vi "TLB Native Dynamic Events ver 0.13.vi"() -> ()   [LabVIEW 2018]
uses:
  Labview Training Phase 2/Enum Controls/States for Action Engine.ctl
  TLB Type Definitions/State Type Definitions, for 0.26g versions and later 2.ctl
  TLB Type Definitions/Intruction Type Definitions.ctl
  TLB Type Definitions/Encoder cluster.ctl
  Experimental VI's/Archived VI's/MOTOR CONTROL NO PID Type Def.ctl
  Underlying VI's/I2C Master VI/I2C MASTER Type Def.ctl
  TLB Type Definitions/PING CLUSTER.ctl
  <vilib>/Studica/Studica Toolkit/NavX/NavX.lvlib
  <vilib>/Studica/Studica Toolkit/Background/DIO Channel.ctl
  Underlying VI's/NavX VI/navX type def.ctl
  <vilib>/myRIO/Instrument Drivers/Utilities/Utilities.lvlib
  <vilib>/Studica/Studica Toolkit/Background/I2C Channel.ctl
  Underlying VI's/I2C Master VI/I2C_MASTER_WRITE_NEW Type Def.ctl
  <vilib>/Studica/Studica Toolkit/NavX/TypeDefs/Flags/Z900_navX_Flags_CalibrationStatusTypeDef.ctl
  <vilib>/Studica/Studica Toolkit/NavX/TypeDefs/Flags/Z900_navX_Flags_OpStatusTypeDef.ctl
panel:
  in  "Latch":bool
  in  "y Stepper value":u8
  out "Arduino Data":T1
  in  "Arduino mode":T2
  out "Detect?":bool
  out "Status":T5 {"OP Status" items=["INITIALIZING", "SELFTEST_IN_PROGRESS", "ERROR", "IMU_AUTOCAL_IN_PROGRESS", "NORMAL"]; "Calibration Status" items=["IMU_CAL_STATE_MASK"=3, "IMU_CAL_STATE_INPROGRESS"=0, "IMU_CAL_STATE_ACCUMULATE"=1, "IMU_CAL_STATE_COMPLETE"=2]}
  out "NavX Readings":T6
  out "TASK ENABLE":bool
  out "Rising Edge":bool
  in  "Green LED":bool
  out "Task Selection":u8
  out "Object detected?":bool
  out "I2C Error":errorcluster
  out "Speed & distance":T7
  out "State Logic":T8=enum."Startup"
  out "elements":T9[](array[typedef])
  in  "STOP TASK":bool
  in  "OK Button":bool
  in  "STOP":bool
  out "error out":errorcluster
  out "Action Queue Items":i32
  out "State Logic Queue Items":i32
  out "Action Queues items":string[](array[string])=["Hardware reset", "Software reset", ""]
  out "Action State":string
  # "TLB FRAMEWORK STATUS"
  # "System Health Status Update"
  # "Test Programme written by Calvin Loke    Dated: 28 Aug 2019\nTest Programme revised by Dr Alex See   Dated 30 Aug 2019\n\nProgramme version:   TLB Native Dynamic Events ver 0.04b.vi"
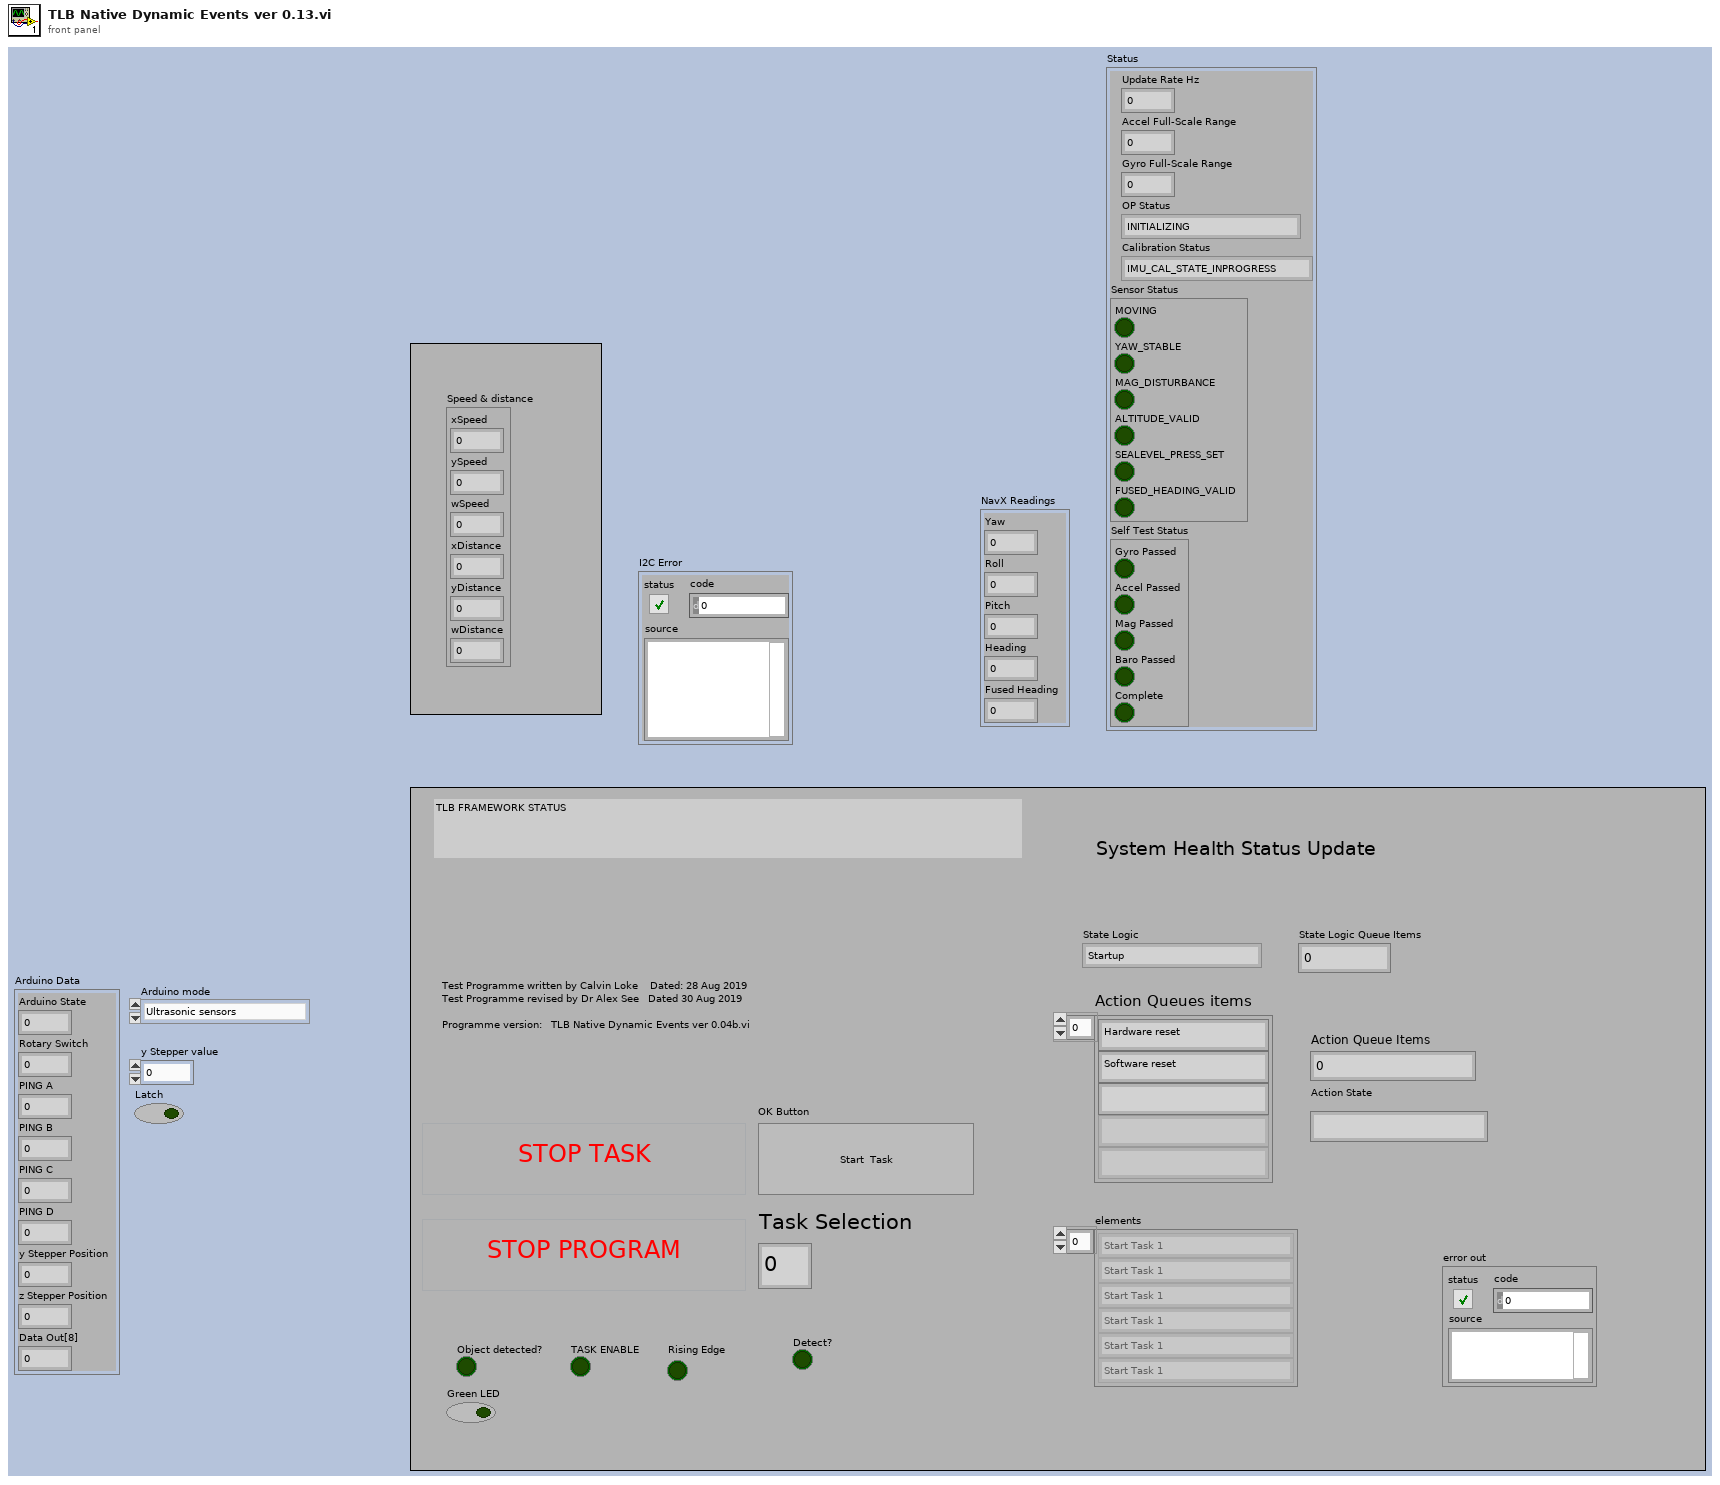
[diagram p1: front panel]
types:
  T1 = cluster{"Arduino State":u8, "Rotary Switch":u8, "PING A":u8, "PING B":u8, "PING C":u8, "PING D":u8, "y Stepper Position":u8, "z Stepper Position":u8, "Data Out[8]":u8}
  T2 = typedef "I2C_MASTER_WRITE_NEW Type Def.ctl" = enum16{"Ultrasonic sensors", "Stepper origin", "zStepper 13.3k", "zStepper 13k", "zStepper 12k", "zStepper 11k", "zStepper 10k", "zStepper 9k", "zStepper 8k", "zStepper 7k", "zStepper 6k", "zStepper 5k", "zStepper 4k", "zStepper 3k", "zStepper 2k", "zStepper 1k", "zStepper 900", "zStepper 800", "zStepper 700", "zStepper 600", "zStepper 500", "zStepper 400", "zStepper 300", "zStepper 200", "zStepper 100", "zStepper 0", "yStepper control", "Open Claw", "Close Claw", "Soft Reset"}
  T3 = typedef "NavX.lvlib/Z900_navX_Flags_OpStatusTypeDef.ctl" = u8
  T4 = typedef "NavX.lvlib/Z900_navX_Flags_CalibrationStatusTypeDef.ctl" = u8
  T5 = cluster{"Update Rate Hz":u8, "Accel Full-Scale Range":u8, "Gyro Full-Scale Range":u16, "OP Status":T3, "Calibration Status":T4, "Sensor Status":cluster{"MOVING":bool, "YAW_STABLE":bool, "MAG_DISTURBANCE":bool, "ALTITUDE_VALID":bool, "SEALEVEL_PRESS_SET":bool, "FUSED_HEADING_VALID":bool}, "Self Test Status":cluster{"Gyro Passed":bool, "Accel Passed":bool, "Mag Passed":bool, "Baro Passed":bool, "Complete":bool}}
  T6 = cluster{"Yaw":dbl, "Roll":dbl, "Pitch":dbl, "Heading":dbl, "Fused Heading":dbl}
  T7 = cluster{"xSpeed":dbl, "ySpeed":dbl, "wSpeed":dbl, "xDistance":dbl, "yDistance":dbl, "wDistance":dbl}
  T8 = typedef "State Type Definitions, for 0.26g versions and later 2.ctl" = enum16{"None", "Startup", "Move to Angle", "True Stop", "Idle", "Shutdown", "Task 1A", "Task 1B", "Task 2:Raise Arm", "Task 2:Sensor Mode", "Task 2:Reverse Mode", "Task 3", "Task 4_A", "Task 4_B", "Task 4_C", "Task 4_D", "Task 5A", "Task 5B", "Task 5C", "Task 5D", "Task 5E: POSITION ARM", "Task 5F: ARM GRAB HEIGHT", "Task 5G: CLOSE CLAW", "Task 5H: RAISE ARM", "Task 6_A", "Task 6_B", "Task 7", "Task 8A: RAISE ARM", "Task 8B: MOVE TO BOX", "Task 8C: CAM BURST", "Task 8D: PROCESS IMAGE", "Task 8E: ROBOT ADJUST", "Task 8F: CAM BURST 2", "Task 8G: PROCESS IMAGE 2", "Task 8H: ARM ADJUST", "Task 8I: ARM GRAB HEIGHT", "Task 8J: CLOSE CLAW", "Task 8K: RAISE MY SWORD", "Task 9A: Raise Arm", "Task 9B: Rotate to Angle", "Task 9C: Detect Box", "Task 9D: MOVE FORWARD", "Task 9E: MOVE LEFT", "Task 9F: SCAN BOX", "Task 9G: MOVE RIGHT", "Task 9H: SCAN BOX 2", "Task 9I: ROTATE 90 CW", "Task 9J: FORWARD", "Task 9K: MOVE RIGHT", "Task 9L: SCAN BOX 3", "Task 9M: MOVE RIGHT", "Task 9N: SCAN BOX 4", "PENIS", "PENIS 2", "PENIS 3", "Task 9R: PROCESS COLOUR", "Task A1: Task 9 Open cam", "Task A2: Task 9 Move Arm", "Task A3: Task 9 Set Timer", "Task A4: Tasl 9 Capture images", "Task A5: Task 9 Close camera", "Task A6: Process Colour", "Task A7: Dispose Camera Buffer"}
  T9 = typedef "Intruction Type Definitions.ctl" = enum16{"None", "Start Task 1", "Start Task 2", "Start Task 3", "Start Task 4", "Start Task 5", "Start Task 6", "Start Task 7", "Start Task 8 - BALL", "Start Task 8 - Gel", "Start Task 8 - Pipe", "Start Task 8 - Soap", "Start Task 9", "Start Task A", "Start Task B", "Exit"}
  T10 = typedef "States for Action Engine.ctl" = enum16{"Initialize", "Write", "Read"}
  T11 = typedef "DIO Channel.ctl" = enum16{"Not Connected", "A/DIO1", "A/DIO2", "A/DIO3", "A/DIO4", "A/DIO5", "A/DIO6", "A/DIO7", "A/DIO13", "B/DIO1", "B/DIO2", "B/DIO3", "B/DIO4", "B/DIO5", "B/DIO6", "B/DIO7", "B/DIO13", "C/DIO0", "C/DIO1", "C/DIO2", "C/DIO3", "C/DIO4", "C/DIO5", "C/DIO6", "C/DIO7"}
  T12 = typedef "PING CLUSTER.ctl" = cluster{"PING_A":u8, "PING_B":u8, "PING_C":u8, "PING_D":u8}
  T13 = typedef "Encoder cluster.ctl" = cluster{"xDistance":dbl, "yDistance":dbl, "wDistance":dbl}
  T14 = typedef "I2C Channel.ctl" = enum16{"Not Connected", "A", "B"}
  T15 = typedef "navX type def.ctl" = enum16{"Get i2C reference", "Read Values", "Zero Yaw"}
  T16 = typedef "State Type Definitions.ctl" = enum16{"None", "Startup", "Move to Angle", "True Stop", "Idle", "Shutdown", "Task 1", "Task 2:Raise Arm", "Task 2:Sensor Mode", "Task 2:Reverse Mode", "Task 3", "Task 4_A", "Task 4_B", "Task 4_C", "Task 4_D", "Task 5A: ARM CAM HEIGHT", "Task 5B: MOVE TO BOX", "Task 5C: CAM BURST", "Task 5D: PROCESS IMAGE", "Task 5E: POSITION ARM", "Task 5F: ARM GRAB HEIGHT", "Task 5G: CLOSE CLAW", "Task 5H: RAISE ARM", "Task 6_A", "Task 6_B", "Task 7", "Task 8A: RAISE ARM", "Task 8B: MOVE TO BOX", "Task 8C: CAM BURST", "Task 8D: PROCESS IMAGE", "Task 8E: ROBOT ADJUST", "Task 8F: CAM BURST 2", "Task 8G: PROCESS IMAGE 2", "Task 8H: ARM ADJUST", "Task 8I: ARM GRAB HEIGHT", "Task 8J: CLOSE CLAW", "Task 8K: RAISE MY SWORD", "Task 9A: Raise Arm", "Task 9B: Rotate to Angle", "Task 9C: Detect Box", "Task 9D: MOVE FORWARD", "Task 9E: MOVE LEFT", "Task 9F: SCAN IMAGE", "Task 9G: PROCESS COLOUR", "Task 9H: MOVE RIGHT", "Task 9I: SCAN IMAGE", "Task 9J: PROCESS COLOUR", "Task 9K: ROTATE 90 CW", "Task 9L: MOVE FORWARD", "Task 9M: MOVE RIGHT", "Task 9N: SCAN IMAGE", "Task 9O: PROCESS COLOUR", "Task 9P: MOVE RIGHT", "Task 9Q: SCAN IMAGE", "Task 9R: PROCESS COLOUR"}
  T17 = typedef "State Type Definitions.ctl" = enum16{"None", "Startup", "Move to Angle", "True Stop", "Idle", "Shutdown", "Task 1", "Task 2", "Task 3", "Task 4_A", "Task 4_B", "Task 4_C", "Task 5", "Task 6", "Task 7", "Task 8", "Task 9", "Task A", "Task B"}
  T18 = typedef "MOTOR CONTROL NO PID Type Def.ctl" = enum16{"Init", "Front Back", "Left Right", "Rotate", "Stop", "Latch"}
  T19 = cluster{"DIO Channel":T11, "FPGA VI Reference Out":refnum<k20>}
  T20 = cluster{"I2C Ref Out":cluster{"I2C Channel":T14, "FPGA VI Reference Out":refnum<k20>}, "Connected":bool, "Slave Address (7-bit)":u8, "Registry":u8[]}
  T21 = typedef "I2C MASTER Type Def.ctl" = enum16{"Last State", "Mode 0", "Mode 1", "Mode 2", "Mode 3", "Mode 4", "Mode 5", "Mode 6", "Mode 7", "Mode 8", "Mode 9", "Mode 10"}
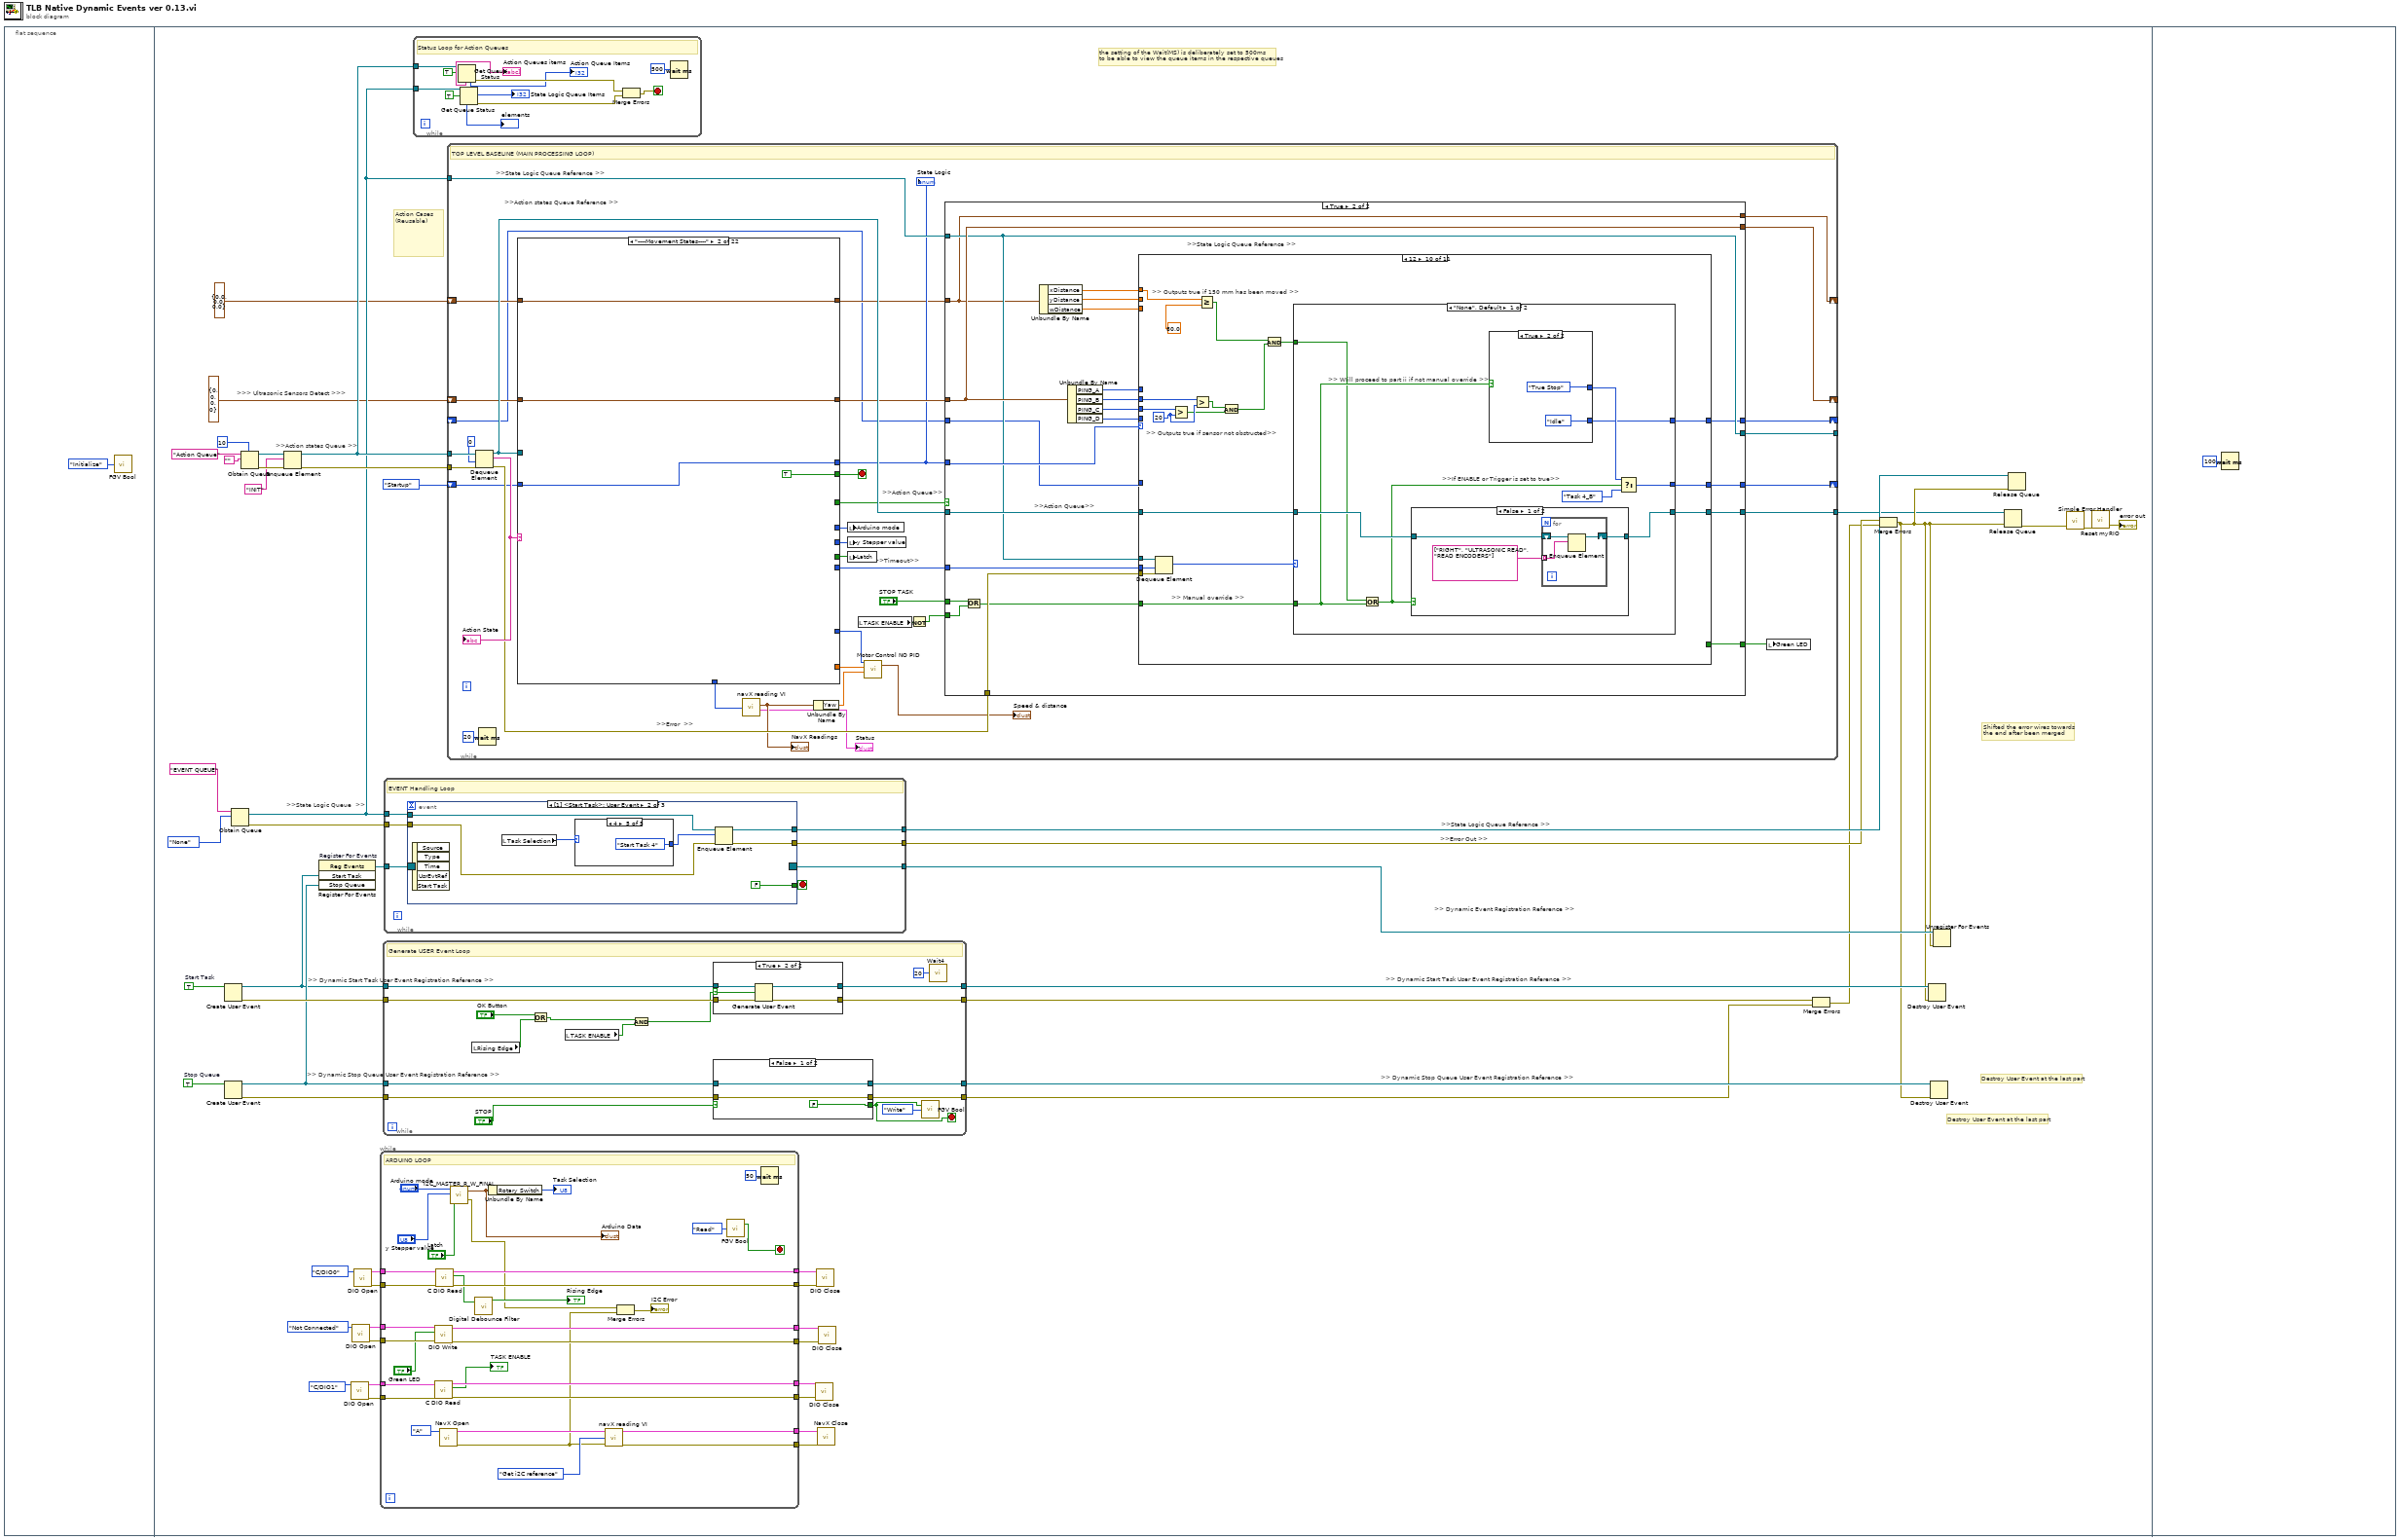
[diagram p0: block diagram]
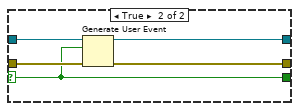
[diagram p2: hidden frame]
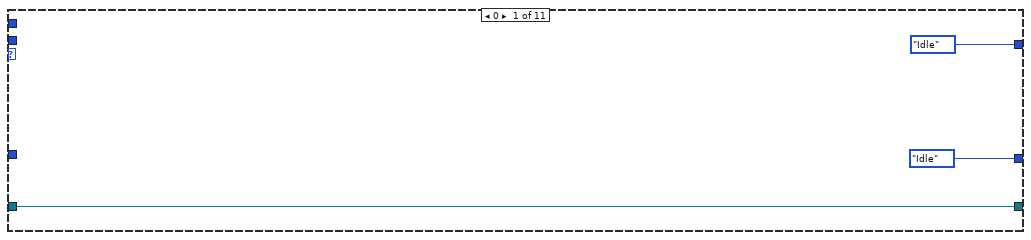
[diagram p5: hidden frame]
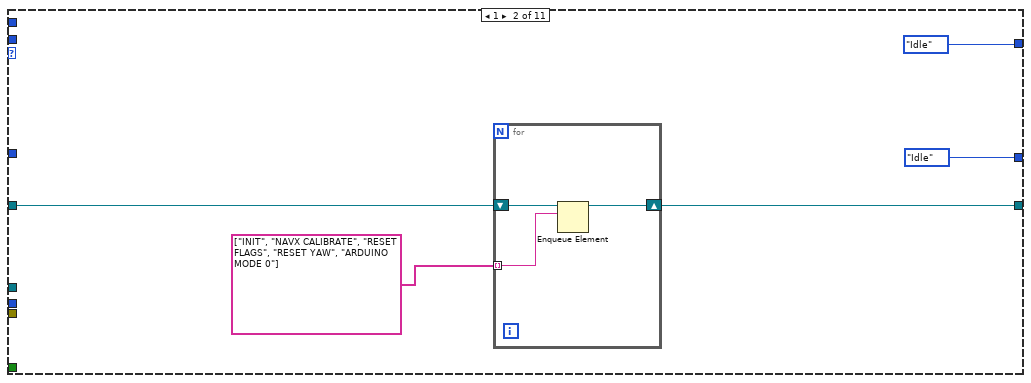
[diagram p6: hidden frame]
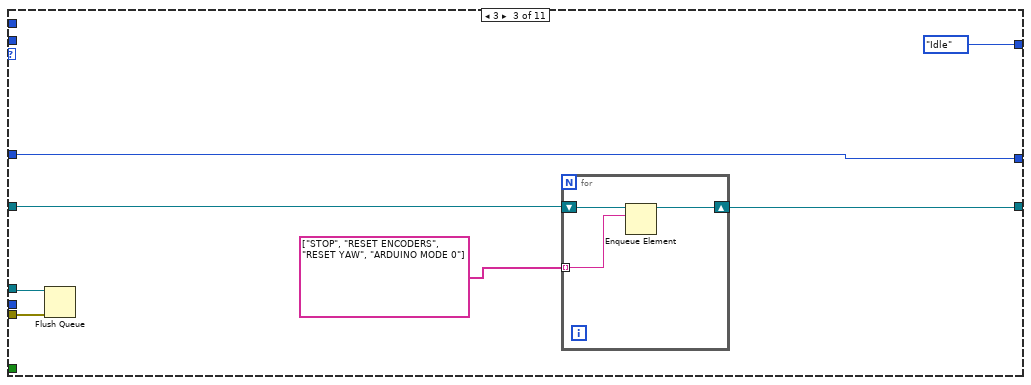
[diagram p7: hidden frame]
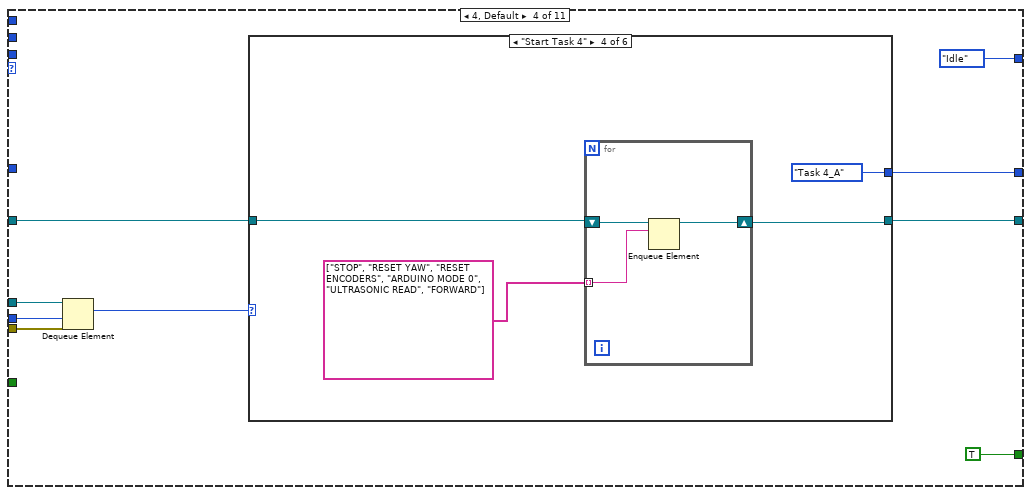
[diagram p8: hidden frame]
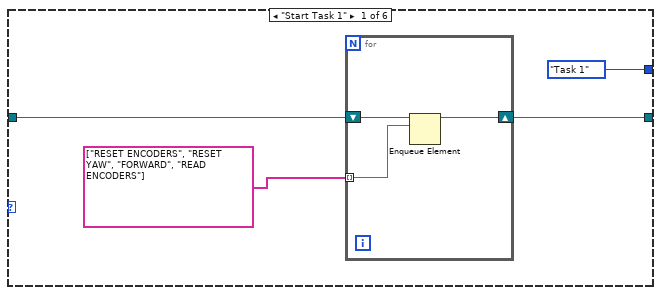
[diagram p9: hidden frame]
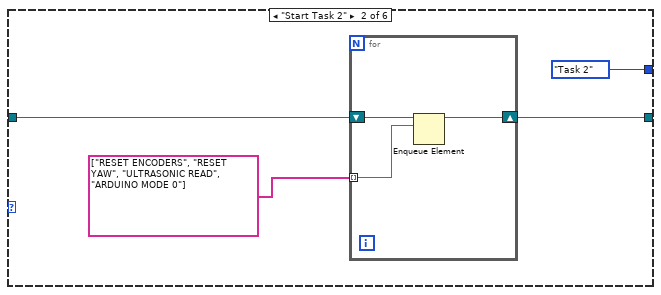
[diagram p10: hidden frame]
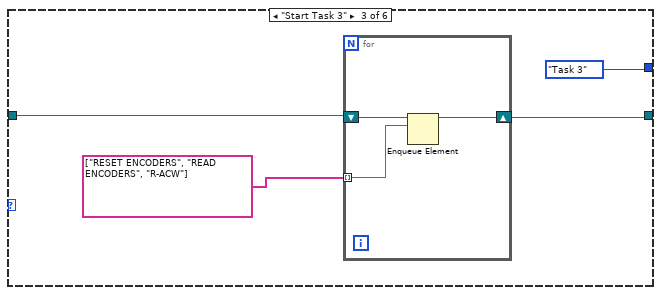
[diagram p11: hidden frame]
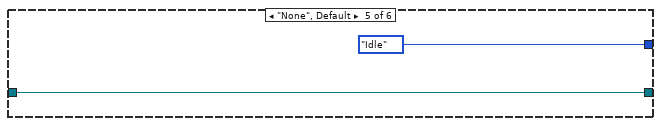
[diagram p12: hidden frame]
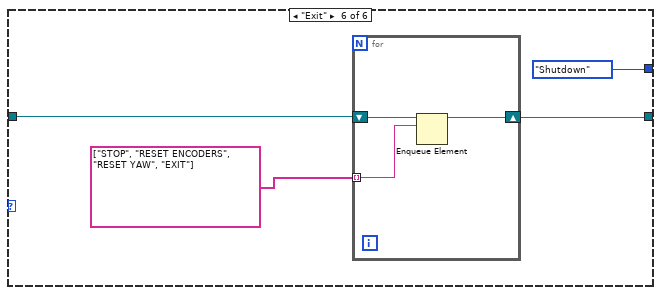
[diagram p13: hidden frame]
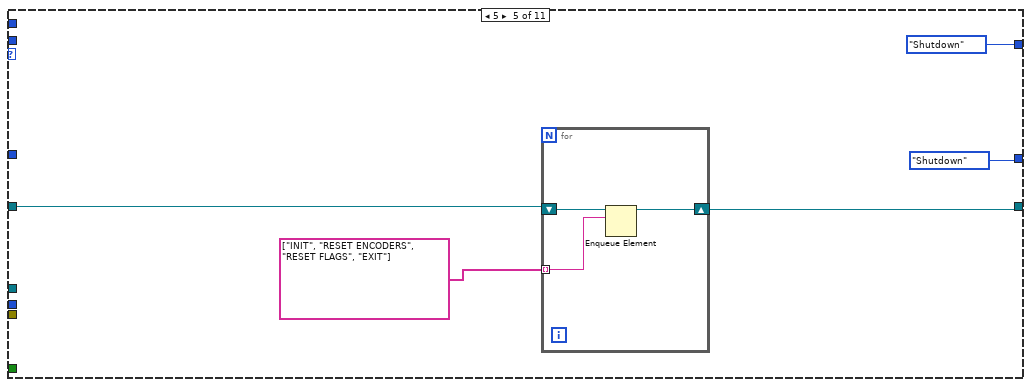
[diagram p14: hidden frame]
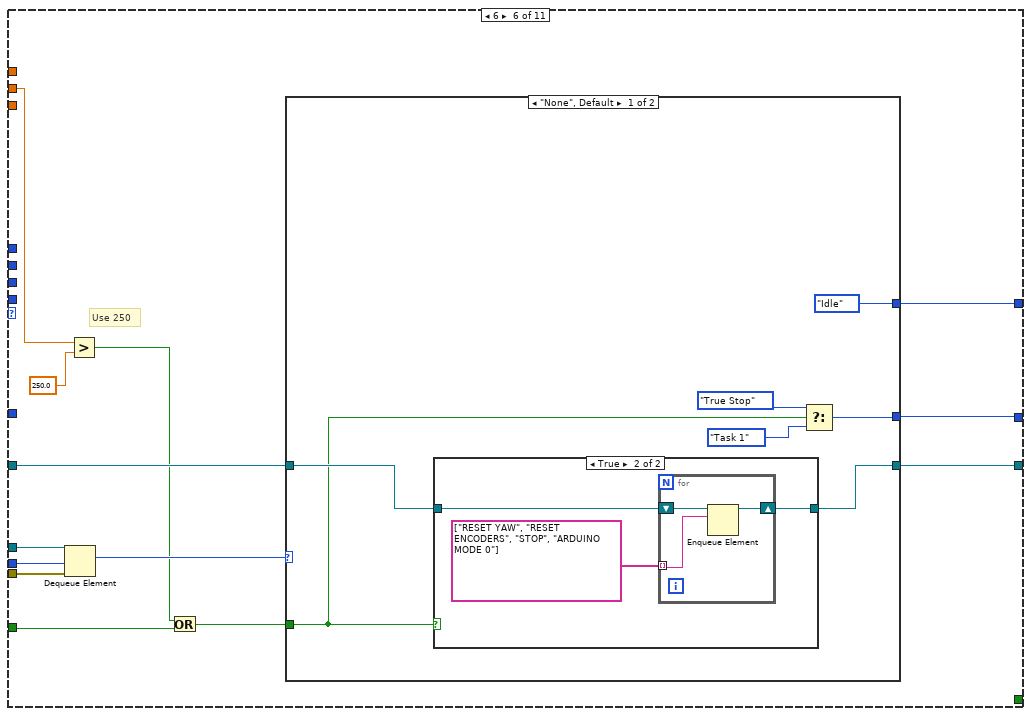
[diagram p15: hidden frame]
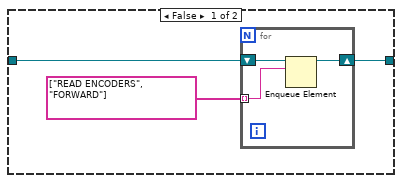
[diagram p16: hidden frame]
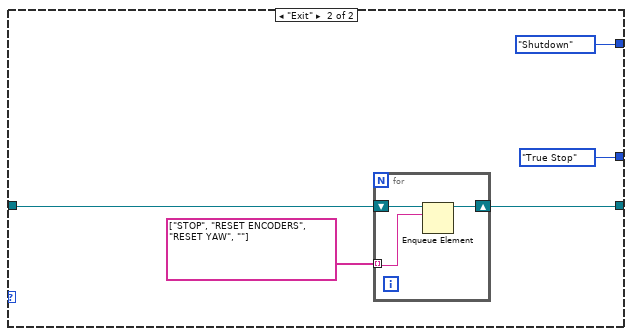
[diagram p17: hidden frame]
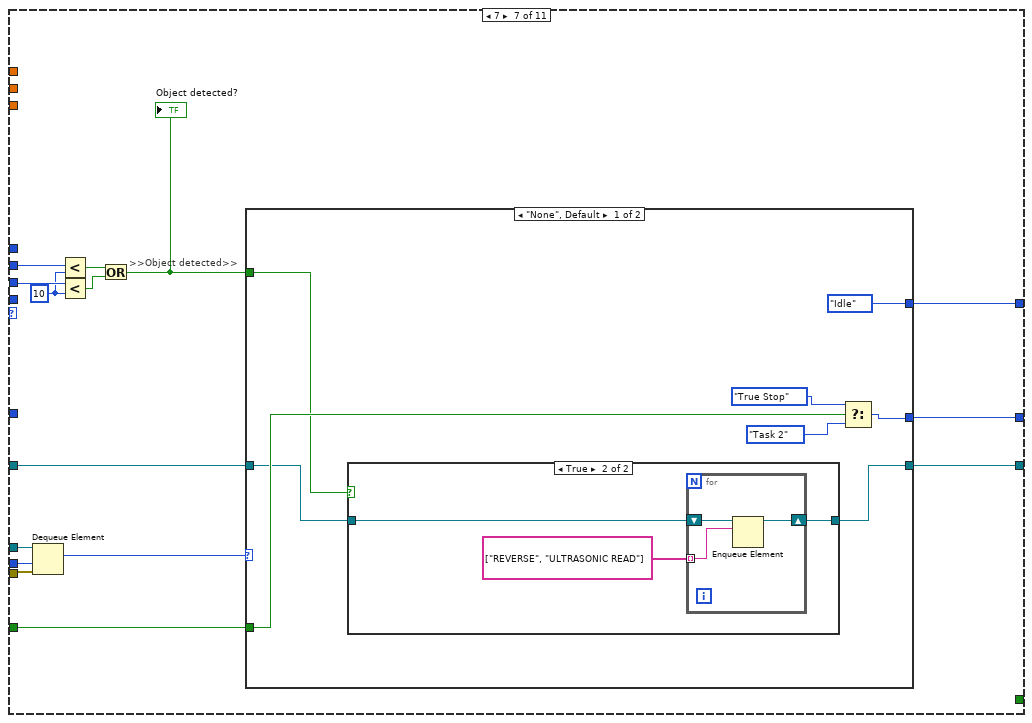
[diagram p18: hidden frame]
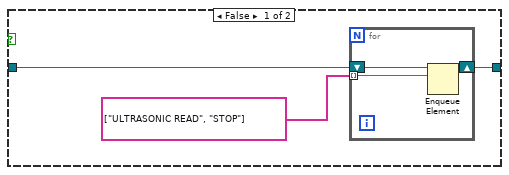
[diagram p19: hidden frame]
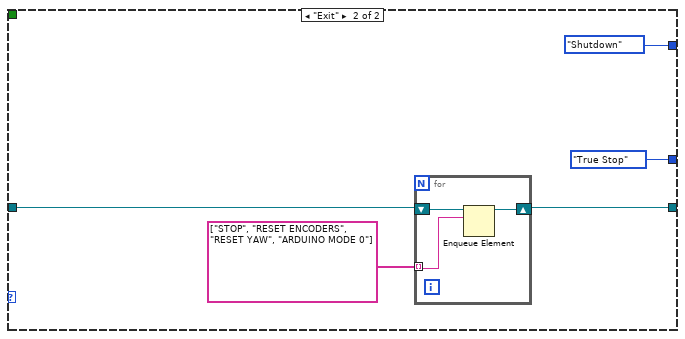
[diagram p20: hidden frame]
diagram:
  n1 = flat-sequence {
    frame #0 {
      n2 = call "FGV Bool.vi"("Init/Read/Write State"=States_for_Action_Engine."Initialize") -> ()  [unwired: 2 in, 2 out]
    }
    frame #1 {
      w53 = TRUE  # Stop Queue
      w52 = TRUE  # Start Task
      # ">>> Ultrasonic Sensors Detect >>>"
      # "the setting of the Wait(MS) is deliberately set to 500ms\nto be able to view the queue items in the respective queues"
      # "Action Cases\n(Reusable)"
      # ">>Error Out >>"
      # ">> Dynamic Stop Queue User Event Registration Reference >>"
      # ">> Dynamic Start Task User Event Registration Reference >>"
      # ">> Dynamic Stop Queue User Event Registration Reference >>"
      # ">> Dynamic Start Task User Event Registration Reference >>"
      # ">> Dynamic Event Registration Reference >>"
      # ">>Action states Queue >>"
      # ">>State Logic Queue  >>"
      # ">>State Logic Queue Reference >>"
      # "Destroy User Event at the last part"
      # "Destroy User Event at the last part"
      # "Shifted the error wires towards\nthe end after been merged"
      n3 = Create User Event(user event datatype=w52) -> (user event=w44:refnum<user-event>, error out=w49:errorcluster)  [unwired: 1 in]
      n4 = Create User Event(user event datatype=w53) -> (user event=w45:refnum<user-event>, error out=w48:errorcluster)  [unwired: 1 in]
      n5 = Obtain Queue(name (unnamed)="EVENT QUEUE", element data type=Intruction_Type_Definitions."None" ("Enum")) -> (queue out=w30:refnum<queue>, error out=w36:errorcluster)  [unwired: 3 in, 1 out]
      n6 = Obtain Queue(max queue size (-1, unlimited)=10, name (unnamed)="Action Queue", element data type="") -> (queue out=w39:refnum<queue>, error out=w35:errorcluster)  [unwired: 2 in, 1 out]
      n7 = Enqueue Element(queue=w39, element="INIT", error in (no error)=w35) -> (queue out=w31:refnum<queue>, error out=w34:errorcluster)  [unwired: 1 in, 1 out]
      n8 = register-events "Register For Events"(w44, w45) -> (reference out=w43:refnum<event-registration>)  [unwired: 2 in, 1 out]
      n9 = call <vilib>:"DIO Open.vi"("DIO Channel"=DIO_Channel."C/DIO1") -> ("error out"=w8:errorcluster, "DIO Info Out"=w9:T19)  [unwired: 9 in]
      n10 = call <vilib>:"DIO Open.vi"("DIO Channel"=DIO_Channel."Not Connected") -> ("error out"=w13:errorcluster, "DIO Info Out"=w15:T19)  [unwired: 9 in]
      n11 = call <vilib>:"DIO Open.vi"("DIO Channel"=DIO_Channel."C/DIO0") -> ("error out"=w18:errorcluster, "DIO Info Out"=w21:T19)  [unwired: 9 in]
      n12 = while {
        tunnel: w21 -> [w81]
        tunnel: [w80] -> w19
        tunnel: w18 -> [w79]
        tunnel: [w78] -> w17
        tunnel: w15 -> [w74]
        tunnel: [w73] -> w14
        tunnel: w13 -> [w72]
        tunnel: [w71] -> w12
        tunnel: [w69] -> w10
        tunnel: w9 -> [w68]
        tunnel: w8 -> [w67]
        tunnel: [w66] -> w7
        tunnel: [w63] -> w6
        tunnel: [w62] -> w5
        stop <- w84 stop-if-true
        # "ARDUINO LOOP"
        n13 = call <vilib>:"DIO Write.vi"("error in (no error)"=w72, "Input"="Green LED", "DIO Info In"=w74) -> ("error out"=w71:errorcluster, "DIO Info Out"=w73:T19)  [unwired: 7 in]
        n14 = call <vilib>:"C DIO Read.vi"("error in (no error)"=w67, "DIO Info In in"=w68) -> ("error out"=w66:errorcluster, "IN"=→"TASK ENABLE":bool, "DIO Info In out"=w69:T19)  [unwired: 7 in]
        n15 = call <vilib>:"C DIO Read.vi"("error in (no error)"=w79, "DIO Info In in"=w81) -> ("error out"=w78:errorcluster, "IN"=w76:bool, "DIO Info In out"=w80:T19)  [unwired: 7 in]
        n16 = call <vilib>:"NavX Open.vi"("I2C Channel"=I2C_Channel."A") -> ("error out"=w60:errorcluster, "NavX Info"=w64:T20)  [unwired: 9 in]
        n17 = call "I2C_MASTER_R_W_FINAL.vi"("Latch"="Latch", "y Stepper value"="y Stepper value", "Arduino mode"="Arduino mode") -> ("error out"=w57:errorcluster, "Arduino Data"=w56:T1)  [unwired: 1 in]
        "Arduino Data" <- w56
        n18 = call "Digital Debounce Filter.vi"("Boolean input"=w76) -> ("Rising Edge"=→"Rising Edge":bool)  [unwired: 1 in, 2 out]
        n19 = Unbundle By Name(w56) -> ("Rotary Switch"=→"Task Selection":u8)
        n20 = call "navX reading VI.vi"("NavX Info In"=w64, "Mode"=navX_type_def."Get i2C reference", "error in (no error)"=w60) -> ("NavX Info Out"=w63:T20, "Error Out"=w62:errorcluster)  [unwired: 2 out]
        n21 = Merge Errors(w57, w60) -> (→"I2C Error":errorcluster)
        n22 = call "FGV Bool.vi"("Init/Read/Write State"=States_for_Action_Engine."Read") -> ("Output node"=w84:bool)  [unwired: 2 in, 1 out]
        n23 = Wait (ms)(milliseconds to wait=u32 50) -> ()  [unwired: 1 out]
      }
      n24 = while {
        tunnel: w44 -> [w114]
        tunnel: w45 -> [w113]
        tunnel: [w112] -> w51
        tunnel: [w111] -> w50
        tunnel: w49 -> [w110]
        tunnel: [w109] -> w47
        tunnel: w48 -> [w108]
        tunnel: [w107] -> w46
        stop <- w105 stop-if-true
        # "Generate USER Event Loop"
        n25 = local read "Rising Edge"() -> (w101:bool)
        n26 = Or(x="OK Button", y=w101) -> (x .or. y?=w100:bool)
        n27 = local read "TASK ENABLE"() -> (w99:bool)
        n28 = And(x=w100, y=w99) -> (x .and. y?=w98:bool)
        n29 = case shown="True" w98 {
          selector: w98 -> [_ w125]
          tunnel: w114 -> [w124 w129]
          tunnel: [w124 w128] -> w111
          tunnel: w110 -> [w123 w127]
          tunnel: [w123 w126] -> w109
          frame False {
          }
          frame True {
            n30 = Generate User Event(user event=w129, event data cluster=w125, error in=w127) -> (user event out=w128:refnum<user-event>, error out=w126:errorcluster)  [unwired: 1 in]
          }
        }
        n31 = case shown="False" "STOP" {
          selector: "STOP" -> [_ w118]
          tunnel: w113 -> [w117 w122]
          tunnel: [w117 w121] -> w112
          tunnel: w108 -> [w116 w120]
          tunnel: [w116 w119] -> w107
          tunnel: [FALSE w118] -> w105
          frame False {
          }
          frame True {
            n32 = Generate User Event(user event=w122, event data cluster=w118, error in=w120) -> (user event out=w121:refnum<user-event>, error out=w119:errorcluster)  [unwired: 1 in]
          }
        }
        n33 = call "FGV Bool.vi"("Init/Read/Write State"=States_for_Action_Engine."Write", "Input Node"=w105) -> ()  [unwired: 1 in, 2 out]
        n34 = call "Wait4"("Count(uSec)"=u32 20) -> ()  [unwired: 1 out]
      }
      n35 = while {
        tunnel: w43 -> [w670]
        tunnel: [w669] -> w42
        tunnel: w30 -> [w667]
        tunnel: [w666] -> w41
        tunnel: w36 -> [w665]
        tunnel: [w664] -> w33
        stop <- w668 stop-if-true
        # "EVENT Handling Loop"
        n36 = event shown="[1] <Start Task>: User Event" {
          selector: w670 -> [_ _ _]
          dyn-events: [_ _ _] -> w669
          timeout: _ -> [_ _ _]
          tunnel: [FALSE FALSE w694] -> w668
          tunnel: w667 -> [w675 w682 w692]
          tunnel: [w674 w681 w693] -> w666
          tunnel: w665 -> [w673 w680 w691]
          tunnel: [w672 w679 w690] -> w664
          event Timeout {
            n37 = event-data() -> ()  [unwired: 1 in, 3 out]
            n38 = Enqueue Element(queue=w675, element=Intruction_Type_Definitions."None" ("Enum"), error in (no error)=w673) -> (queue out=w674:refnum<queue>, error out=w672:errorcluster)  [unwired: 1 in, 1 out]
          }
          event User Event {
            n39 = event-data() -> ()  [unwired: 1 in, 5 out]
            n40 = local read "Task Selection"() -> (w677:u8)
            n41 = case shown="4" w677 {
              tunnel: [Intruction_Type_Definitions."None" ("Enum") Intruction_Type_Definitions."Start Task 1" ("Enum") Intruction_Type_Definitions."Start Task 2" ("Enum") Intruction_Type_Definitions."Start Task 3" ("Enum") Intruction_Type_Definitions."Start Task 4" ("Enum")] -> w678
              frame 0, Default {
              }
              frame 1 {
              }
              frame 2 {
              }
              frame 3 {
              }
              frame 4 {
              }
            }
            n42 = Enqueue Element(queue=w682, element=w678, error in (no error)=w680) -> (queue out=w681:refnum<queue>, error out=w679:errorcluster)  [unwired: 1 in, 1 out]
          }
          event User Event {
            n43 = event-data() -> ("Stop Queue"=w694:bool)  [unwired: 1 in, 4 out]
            n44 = Enqueue Element At Opposite End(queue=w692, element=Intruction_Type_Definitions."Exit" ("Enum"), error in (no error)=w691) -> (queue out=w693:refnum<queue>, error out=w690:errorcluster)  [unwired: 1 in, 1 out]
          }
        }
      }
      n45 = while {
        tunnel: w31 -> [w95]
        tunnel: w30 -> [w92]
        stop <- w89 stop-if-true
        # "Status Loop for Action Queues"
        n46 = Get Queue Status(queue=w95, return elements? (F)=TRUE) -> (error out=w91:errorcluster, # elements in queue=→"Action Queue Items":i32, elements=→"Action Queues items":string[])  [unwired: 1 in, 5 out]
        n47 = Get Queue Status(queue=w92, return elements? (F)=TRUE) -> (# pending remove=→"State Logic Queue Items":i32, error out=w90:errorcluster, elements=→"elements":T9[])  [unwired: 1 in, 5 out]
        n48 = Merge Errors(w91, w90) -> (w89:errorcluster)
        n49 = Wait (ms)(milliseconds to wait=u32 500) -> ()  [unwired: 1 out]
      }
      n50 = while {
        tunnel: w30 -> [w155]
        tunnel: w31 -> [w167]
        tunnel: w34 -> [w165]
        tunnel: [w164] -> _
        tunnel: [w163] -> w24
        shift-right: [w156] -> _
        shift-left: T12 {"PING_A"=0, "PING_B"=0, "PING_C"=0, "PING_D"=0} -> [w158]
        shift-right: [w149] -> _
        shift-left: State_Type_Definitions,_for_0.26g_versions_and_later_2."Startup" ("Enum") -> [w152]
        shift-right: [w145] -> _
        shift-left: T13 {"xDistance"=0.0, "yDistance"=0.0, "wDistance"=0.0} -> [w147]
        shift-right: [w139] -> _
        shift-left: _ -> [w138]
        stop <- w154 stop-if-true
        # ">>Error  >>"
        # ">>Action Queue>>"
        # ">>Timeout>>"
        # ">>Action states Queue Reference >>"
        # ">>State Logic Queue Reference >>"
        # "TOP LEVEL BASELINE (MAIN PROCESSING LOOP)"
        n51 = Dequeue Element(queue=w167, timeout in ms (-1)=0, error in (no error)=w165) -> (queue out=w159:refnum<queue>, element=w166:string, error out=w160:errorcluster)  [unwired: 1 out]
        "Action State" <- w166
        n52 = Wait (ms)(milliseconds to wait=u32 20) -> ()  [unwired: 1 out]
        n53 = case shown="\"----Movement States----\"" w166 {
          tunnel: [_ _ _ _ _ _ _ _ _ _ _ _ _ _ _ _ 0 w641 _ _ _ _] -> w162
          tunnel: w159 -> [_ _ _ _ _ _ _ _ _ _ _ _ _ _ _ _ _ _ _ _ _ _]
          tunnel: w158 -> [w543 w547 w553 w558 w563 w567 w573 w579 w584 w586 w597 w608 w611 w620 w623 w626 w633 w642 w646 w650 w656 w663]
          tunnel: [w543 w547 w553 w558 w563 w567 w573 w579 w584 w586 w597 w609 w611 w621 w623 w626 w633 w642 w646 w650 w655 w663] -> w157
          tunnel: [TRUE TRUE _ _ _ _ _ _ _ _ _ _ _ _ _ _ _ _ _ _ _ _] -> w154
          tunnel: w152 -> [w541 w545 w552 w557 w562 w566 w572 w578 w583 w585 w596 w607 w610 w619 w622 w625 w630 w639 w645 w649 w654 w662]
          tunnel: [_ _ _ _ _ _ _ _ _ _ _ _ _ _ _ _ _ TRUE _ _ _ _] -> w151
          tunnel: [w541 w545 w552 w557 w562 w566 w572 w578 w583 w585 w596 w607 w610 w619 w622 w625 w630 w639 w645 w649 w654 w662] -> w150
          tunnel: w147 -> [w540 w544 w551 w556 w561 w565 w571 w577 w582 w587 w595 w606 w612 w618 w624 w627 w629 w638 w647 w651 w653 w661]
          tunnel: [w540 w544 w551 w556 w561 w565 w571 w577 w582 w587 w594 w606 w612 w617 w624 w627 w629 w638 w647 w651 w653 w661] -> w146
          tunnel: [_ _ 0.4 ("Speed") -0.3 ("Speed") 0.19999999999999998 ("Speed") -0.2 ("Speed") _ 0.3 ("Speed") -0.5 ("Speed") _ _ _ _ 0.0 ("Speed") _ _ _ _ _ _ _ _] -> w144
          tunnel: [_ _ MOTOR_CONTROL_NO_PID_Type_Def."Front Back" ("Direction") _ MOTOR_CONTROL_NO_PID_Type_Def."Rotate" ("Direction") _ MOTOR_CONTROL_NO_PID_Type_Def."Stop" ("Direction") MOTOR_CONTROL_NO_PID_Type_Def."Left Right" ("Direction") MOTOR_CONTROL_NO_PID_Type_Def."Front Back" ("Direction") _ MOTOR_CONTROL_NO_PID_Type_Def."Latch" ("Direction") MOTOR_CONTROL_NO_PID_Type_Def."Latch" ("Direction") _ _ _ _ _ MOTOR_CONTROL_NO_PID_Type_Def."Latch" ("Direction") _ MOTOR_CONTROL_NO_PID_Type_Def."Init" ("Direction") _ MOTOR_CONTROL_NO_PID_Type_Def."Init" ("Direction")] -> w142
          tunnel: [_ _ navX_type_def."Read Values" ("Mode") navX_type_def."Read Values" ("Mode") _ _ navX_type_def."Read Values" ("Mode") navX_type_def."Read Values" ("Mode") _ _ navX_type_def."Read Values" ("Mode") navX_type_def."Read Values" ("Mode") _ navX_type_def."Zero Yaw" ("Mode") _ _ navX_type_def."Zero Yaw" ("Mode") navX_type_def."Read Values" ("Mode") _ _ _ navX_type_def."Zero Yaw" ("Mode")] -> w136
          tunnel: [_ _ _ _ _ _ _ _ _ _ _ I2C_MASTER_WRITE_NEW_Type_Def."Ultrasonic sensors" ("Arduino mode") _ _ _ _ _ _ _ _ _ _] -> w132
          tunnel: [_ _ _ _ _ _ _ _ _ _ _ _ _ _ _ _ _ TRUE ("Latch") _ _ _ _] -> w131
          tunnel: [_ _ _ _ _ _ _ _ _ _ _ _ _ _ _ _ _ u8 0 ("y Stepper value") _ _ _ _] -> w130
          frame "Exit" {
          }
          frame "----Movement States----" {
          }
          frame "FORWARD" {
          }
          frame "LEFT" {
            (unwired) I2C_MASTER_Type_Def."Last State" ("Arduino Mode")
          }
          frame "R-ACW" {
            (unwired) I2C_MASTER_Type_Def."Last State" ("Arduino Mode")
          }
          frame "R-CW" {
            (unwired) I2C_MASTER_Type_Def."Last State" ("Arduino Mode")
          }
          frame "STOP" {
            (unwired) I2C_MASTER_Type_Def."Last State" ("Arduino Mode")
            n54 = Wait (ms)(milliseconds to wait=u32 200) -> ()  [unwired: 1 out]
          }
          frame "RIGHT" {
            (unwired) I2C_MASTER_Type_Def."Last State" ("Arduino Mode")
          }
          frame "REVERSE" {
            (unwired) I2C_MASTER_Type_Def."Last State" ("Arduino Mode")
          }
          frame "----SENSOR READING---- " {
            (unwired) I2C_MASTER_Type_Def."Last State" ("Arduino Mode")
          }
          frame "READ ENCODERS" {
            (unwired) I2C_MASTER_Type_Def."Last State" ("Arduino Mode")
            # ">>> Current encoder distance >>>"
            # ">>> Ultrasonic Sensors Detect >>>"
            n55 = local read "Speed & distance"() -> (w593:T7)
            n56 = Unbundle By Name(w593) -> ("xDistance"=w592:dbl, "yDistance"=w591:dbl, "wDistance"=w590:dbl)
            n57 = Bundle By Name(cluster=w595, "xDistance"=w592, "yDistance"=w591, "wDistance"=w590) -> (w594:T13)
          }
          frame "ULTRASONIC READ" {
            # "Object detection"
            n58 = local read "Arduino Data"() -> (w603:T1)
            n59 = Unbundle By Name(w603) -> ("PING A"=w602:u8, "PING B"=w601:u8, "PING C"=w600:u8, "PING D"=w599:u8)
            n60 = Bundle By Name(cluster=w608, "PING_A"=w602, "PING_B"=w601, "PING_C"=w600, "PING_D"=w599) -> (w609:T12)
          }
          frame "----SYSTEM MODES----" {
            (unwired) I2C_MASTER_Type_Def."Last State" ("Arduino Mode")
          }
          frame "INIT" {
            (unwired) I2C_MASTER_Type_Def."Last State" ("Arduino Mode")
            w614 = 0
            w616 = 0.0
            # ">>State Logic  >>"
            n61 = Bundle By Name(cluster=w620, "PING_A"=w614, "PING_B"=w614, "PING_C"=w614, "PING_D"=w614) -> (w621:T12)
            n62 = Bundle By Name(cluster=w618, "xDistance"=w616, "yDistance"=w616, "wDistance"=w616) -> (w617:T13)
          }
          frame "ARDUINO MODE 0" {
            (unwired) I2C_MASTER_Type_Def."Mode 0" ("Arduino Mode")
          }
          frame "ARDUINO MODE 1" {
            (unwired) I2C_MASTER_Type_Def."Mode 1" ("Arduino Mode")
          }
          frame "NAVX CALIBRATE" {
            (unwired) I2C_MASTER_Type_Def."Last State" ("Arduino Mode")
            # "Adds a 15 second delay to the startup process \nfor the NavX to calibrate"
            n63 = Wait (ms)(milliseconds to wait=u32 5000) -> ()  [unwired: 1 out]
          }
          frame "NO ACTION", Default {
            n64 = case shown="4" w639 {
              tunnel: [0 100] -> w641
              frame 1, Default {
              }
              frame 4 {
              }
            }
          }
          frame "----RESET CASES----" {
            (unwired) I2C_MASTER_Type_Def."Last State" ("Arduino Mode")
          }
          frame "RESET ENCODERS" {
            (unwired) I2C_MASTER_Type_Def."Last State" ("Arduino Mode")
          }
          frame "RESET FLAGS" {
            (unwired) I2C_MASTER_Type_Def."Last State" ("Arduino Mode")
            w652 = 0
            # "Resets any software variables\nand/or non-critical states"
            n65 = Wait (ms)(milliseconds to wait=u32 20) -> ()  [unwired: 1 out]
            n66 = Bundle By Name(cluster=w656, "PING_A"=w652, "PING_B"=w652, "PING_C"=w652, "PING_D"=w652) -> (w655:T12)
          }
          frame "RESET YAW" {
            (unwired) I2C_MASTER_Type_Def."Last State" ("Arduino Mode")
            n67 = Wait (ms)(milliseconds to wait=u32 100) -> ()  [unwired: 1 out]
          }
        }
        "State Logic" <- w150
        n68 = call "navX reading VI.vi"("Mode"=w136) -> ("NavX Readings"=w137:T6, "Status"=→"Status":T5)  [unwired: 2 in, 2 out]
        "NavX Readings" <- w137
        n69 = Unbundle By Name(w137) -> ("Yaw"=w135:dbl)
        n70 = local write "Arduino mode"(w132) -> ()
        n71 = local write "y Stepper value"(w130) -> ()
        n72 = local write "Latch"(w131) -> ()
        n73 = local read "TASK ENABLE"() -> (w141:bool)
        n74 = call "Motor Control NO PID.vi"("Yaw"=w135, "Speed"=w144, "Direction"=w142) -> ("Speed & distance"=→"Speed & distance":T7)  [unwired: 1 in, 1 out]
        n75 = Not(x=w141) -> (.not. x?=w140:bool)
        n76 = case shown="True" w151 {
          tunnel: w155 -> [w173 w190]
          tunnel: w159 -> [w169 w192]
          tunnel: [w173 w190] -> w164
          tunnel: [w169 w193] -> w163
          tunnel: w160 -> [_ w188]
          tunnel: w162 -> [_ w189]
          tunnel: w157 -> [w172 w195]
          tunnel: [w172 w195] -> w156
          tunnel: "STOP TASK" -> [_ w178]
          tunnel: w150 -> [w171 w194]
          tunnel: [w171 w191] -> w149
          tunnel: w146 -> [w170 w184]
          tunnel: [w170 w184] -> w145
          tunnel: w140 -> [_ w179]
          tunnel: [w168 w176] -> w139
          tunnel: w138 -> [w168 w175]
          tunnel: [_ w174] -> w133
          frame False {
          }
          frame True {
            # ">>Action Queue>>"
            # ">>State Logic Queue Reference >>"
            n77 = Or(x=w178, y=w179) -> (x .or. y?=w177:bool)
            n78 = Unbundle By Name(w184) -> ("xDistance"=w181:dbl, "yDistance"=w182:dbl, "wDistance"=w183:dbl)
            n79 = Unbundle By Name(w195) -> ("PING_A"=w187:u8, "PING_B"=w186:u8, "PING_C"=w185:u8, "PING_D"=w180:u8)
            n80 = case shown="12" w194 {
              tunnel: [w197 w200 w211 w219 w264 w276 w312 w358 w402 w459 w496] -> w193
              tunnel: w192 -> [w197 w203 w212 w222 w266 w277 w313 w359 w408 w452 w500]
              tunnel: [State_Type_Definitions,_for_0.26g_versions_and_later_2."Idle" ("Enum") State_Type_Definitions,_for_0.26g_versions_and_later_2."Idle" ("Enum") w207 w221 State_Type_Definitions,_for_0.26g_versions_and_later_2."Shutdown" ("Enum") w278 w315 w357 w403 w458 w497] -> w191
              tunnel: w190 -> [_ _ w210 w225 _ w283 w325 w366 w407 w456 w501]
              tunnel: w189 -> [_ _ _ w224 _ w282 w324 w365 w406 w455 w493]
              tunnel: w188 -> [_ _ w209 w220 _ w281 w323 w364 w405 w454 w492]
              tunnel: w177 -> [_ _ _ _ _ w275 w314 w361 w401 w457 w498]
              tunnel: w187 -> [_ _ _ _ _ _ _ _ _ _ _]
              tunnel: w186 -> [_ _ _ _ _ _ w321 _ w399 w447 w503]
              tunnel: w185 -> [_ _ _ _ _ _ w320 _ w400 w448 w502]
              tunnel: w183 -> [_ _ _ _ _ _ _ w363 _ _ _]
              tunnel: w182 -> [_ _ _ _ _ w274 _ _ _ _ _]
              tunnel: w181 -> [_ _ _ _ _ _ _ _ _ w443 _]
              tunnel: w180 -> [_ _ _ _ _ _ _ _ _ _ _]
              tunnel: [State_Type_Definitions,_for_0.26g_versions_and_later_2."Idle" ("Enum") State_Type_Definitions,_for_0.26g_versions_and_later_2."Idle" ("Enum") State_Type_Definitions,_for_0.26g_versions_and_later_2."Idle" ("Enum") State_Type_Definitions,_for_0.26g_versions_and_later_2."Idle" ("Enum") State_Type_Definitions,_for_0.26g_versions_and_later_2."Shutdown" ("Enum") w271 w311 w354 w394 w442 w495] -> w176
              tunnel: w175 -> [_ _ w207 _ _ _ _ _ _ _ _]
              tunnel: [_ _ _ TRUE ("Green LED") _ _ _ _ _ _ _] -> w174
              frame 0 {
              }
              frame 1 {
                n81 = for {
                  shift-right: [w206] -> w200
                  shift-left: w203 -> [w205]
                  tunnel: string[] ["INIT", "NAVX CALIBRATE", "RESET FLAGS", "RESET YAW", "ARDUINO MODE 0"] -> [w204] mode=indexing
                  n82 = Enqueue Element(queue=w205, element=w204) -> (queue out=w206:refnum<queue>)  [unwired: 2 in, 2 out]
                }
              }
              frame 3 {
                n83 = Flush Queue(queue=w210, error in (no error)=w209) -> ()  [unwired: 3 out]
                n84 = for {
                  shift-right: [w216] -> w211
                  shift-left: w212 -> [w215]
                  tunnel: string[] ["STOP", "RESET ENCODERS", "RESET YAW", "ARDUINO MODE 0"] -> [w214] mode=indexing
                  n85 = Enqueue Element(queue=w215, element=w214) -> (queue out=w216:refnum<queue>)  [unwired: 2 in, 2 out]
                }
              }
              frame 4, Default {
                n86 = Dequeue Element(queue=w225, timeout in ms (-1)=w224, error in (no error)=w220) -> (element=w223:T9)  [unwired: 3 out]
                n87 = case shown="\"Start Task 4\"" w223 {
                  tunnel: [w227 w234 w241 w248 w255 w257] -> w219
                  tunnel: w222 -> [w228 w235 w242 w249 w255 w258]
                  tunnel: [State_Type_Definitions."Task 1" ("Enum") State_Type_Definitions."Task 2" ("Enum") State_Type_Definitions,_for_0.26g_versions_and_later_2."Task 3" ("Enum") State_Type_Definitions,_for_0.26g_versions_and_later_2."Task 4_A" ("Enum") State_Type_Definitions,_for_0.26g_versions_and_later_2."Idle" ("Enum") State_Type_Definitions,_for_0.26g_versions_and_later_2."Shutdown" ("Enum")] -> w221
                  frame "Start Task 1" {
                    n88 = for {
                      shift-right: [w232] -> w227
                      shift-left: w228 -> [w231]
                      tunnel: string[] ["RESET ENCODERS", "RESET YAW", "FORWARD", "READ ENCODERS"] -> [w230] mode=indexing
                      n89 = Enqueue Element(queue=w231, element=w230) -> (queue out=w232:refnum<queue>)  [unwired: 2 in, 2 out]
                    }
                  }
                  frame "Start Task 2" {
                    n90 = for {
                      shift-right: [w239] -> w234
                      shift-left: w235 -> [w238]
                      tunnel: string[] ["RESET ENCODERS", "RESET YAW", "ULTRASONIC READ", "ARDUINO MODE 0"] -> [w237] mode=indexing
                      n91 = Enqueue Element(queue=w238, element=w237) -> (queue out=w239:refnum<queue>)  [unwired: 2 in, 2 out]
                    }
                  }
                  frame "Start Task 3" {
                    n92 = for {
                      shift-right: [w246] -> w241
                      shift-left: w242 -> [w245]
                      tunnel: string[] ["RESET ENCODERS", "READ ENCODERS", "R-ACW"] -> [w244] mode=indexing
                      n93 = Enqueue Element(queue=w245, element=w244) -> (queue out=w246:refnum<queue>)  [unwired: 2 in, 2 out]
                    }
                  }
                  frame "Start Task 4" {
                    n94 = for {
                      shift-right: [w253] -> w248
                      shift-left: w249 -> [w252]
                      tunnel: string[] ["STOP", "RESET YAW", "RESET ENCODERS", "ARDUINO MODE 0", "ULTRASONIC READ", "FORWARD"] -> [w251] mode=indexing
                      n95 = Enqueue Element(queue=w252, element=w251) -> (queue out=w253:refnum<queue>)  [unwired: 2 in, 2 out]
                    }
                  }
                  frame "None", Default {
                  }
                  frame "Exit" {
                    n96 = for {
                      shift-right: [w262] -> w257
                      shift-left: w258 -> [w261]
                      tunnel: string[] ["STOP", "RESET ENCODERS", "RESET YAW", "EXIT"] -> [w260] mode=indexing
                      n97 = Enqueue Element(queue=w261, element=w260) -> (queue out=w262:refnum<queue>)  [unwired: 2 in, 2 out]
                    }
                  }
                }
              }
              frame 5 {
                n98 = for {
                  shift-right: [w270] -> w264
                  shift-left: w266 -> [w269]
                  tunnel: string[] ["INIT", "RESET ENCODERS", "RESET FLAGS", "EXIT"] -> [w268] mode=indexing
                  n99 = Enqueue Element(queue=w269, element=w268) -> (queue out=w270:refnum<queue>)  [unwired: 2 in, 2 out]
                }
              }
              frame 6 {
                # "Use 250"
                n100 = Dequeue Element(queue=w283, timeout in ms (-1)=w282, error in (no error)=w281) -> (element=w280:T9)  [unwired: 3 out]
                n101 = Greater?(x=w274, y=250.0) -> (0:w272:bool)
                n102 = Or(x=w272, y=w275) -> (x .or. y?=w279:bool)
                n103 = case shown="\"None\", Default" w280 {
                  tunnel: w279 -> [w286 _]
                  tunnel: [w290 State_Type_Definitions,_for_0.26g_versions_and_later_2."True Stop" ("Enum")] -> w278
                  tunnel: w277 -> [w287 w305]
                  tunnel: [w285 w304] -> w276
                  tunnel: [State_Type_Definitions,_for_0.26g_versions_and_later_2."Idle" ("Enum") State_Type_Definitions,_for_0.26g_versions_and_later_2."Shutdown" ("Enum")] -> w271
                  frame "None", Default {
                    n104 = case shown="True" w286 {
                      tunnel: w287 -> [w293 w299]
                      tunnel: [w292 w297] -> w285
                      frame False {
                        n105 = for {
                          shift-right: [w295] -> w292
                          shift-left: w293 -> [w296]
                          tunnel: string[] ["READ ENCODERS", "FORWARD"] ("element") -> [w294] mode=indexing
                          n106 = Enqueue Element(queue=w296, element=w294) -> (queue out=w295:refnum<queue>)  [unwired: 2 in, 2 out]
                        }
                      }
                      frame True {
                        n107 = for {
                          shift-right: [w301] -> w297
                          shift-left: w299 -> [w302]
                          tunnel: string[] ["RESET YAW", "RESET ENCODERS", "STOP", "ARDUINO MODE 0"] -> [w300] mode=indexing
                          n108 = Enqueue Element(queue=w302, element=w300) -> (queue out=w301:refnum<queue>)  [unwired: 2 in, 2 out]
                        }
                      }
                    }
                    n109 = Select(t=State_Type_Definitions,_for_0.26g_versions_and_later_2."True Stop" ("Enum"), s=w286, f=State_Type_Definitions."Task 1" ("Enum")) -> (s? t:f=w290:u16)
                  }
                  frame "Exit" {
                    n110 = for {
                      shift-right: [w309] -> w304
                      shift-left: w305 -> [w310]
                      tunnel: string[] ["STOP", "RESET ENCODERS", "RESET YAW", ""] -> [w308] mode=indexing
                      n111 = Enqueue Element(queue=w310, element=w308) -> (queue out=w309:refnum<queue>)  [unwired: 2 in, 2 out]
                    }
                  }
                }
              }
              frame 7 {
                w319 = u16 10 ("y")
                # ">>Object detected>>"
                n112 = Dequeue Element(queue=w325, timeout in ms (-1)=w324, error in (no error)=w323) -> (element=w322:T9)  [unwired: 3 out]
                n113 = Less?(x=w321, y=w319) -> (x < y?=w318:bool)
                n114 = Less?(x=w320, y=w319) -> (x < y?=w317:bool)
                n115 = Or(x=w318, y=w317) -> (x .or. y?=w316:bool)
                "Object detected?" <- w316
                n116 = case shown="\"None\", Default" w322 {
                  tunnel: w316 -> [w329 _]
                  tunnel: [w331 State_Type_Definitions,_for_0.26g_versions_and_later_2."True Stop" ("Enum")] -> w315
                  tunnel: w314 -> [w330 _]
                  tunnel: w313 -> [w328 w348]
                  tunnel: [w327 w349] -> w312
                  tunnel: [State_Type_Definitions,_for_0.26g_versions_and_later_2."Idle" ("Enum") State_Type_Definitions,_for_0.26g_versions_and_later_2."Shutdown" ("Enum")] -> w311
                  frame "None", Default {
                    n117 = case shown="True" w329 {
                      tunnel: w328 -> [w335 w342]
                      tunnel: [w336 w341] -> w327
                      frame False {
                        n118 = for {
                          tunnel: string[] ["ULTRASONIC READ", "STOP"] ("element") -> [w337] mode=indexing
                          shift-right: [w339] -> w336
                          shift-left: w335 -> [w338]
                          n119 = Enqueue Element(queue=w338, element=w337) -> (queue out=w339:refnum<queue>)  [unwired: 2 in, 2 out]
                        }
                      }
                      frame True {
                        n120 = for {
                          shift-right: [w344] -> w341
                          shift-left: w342 -> [w345]
                          tunnel: string[] ["REVERSE", "ULTRASONIC READ"] -> [w343] mode=indexing
                          n121 = Enqueue Element(queue=w345, element=w343) -> (queue out=w344:refnum<queue>)  [unwired: 2 in, 2 out]
                        }
                      }
                    }
                    n122 = Select(t=State_Type_Definitions,_for_0.26g_versions_and_later_2."True Stop" ("Enum"), s=w330, f=State_Type_Definitions."Task 2" ("Enum")) -> (s? t:f=w331:u16)
                  }
                  frame "Exit" {
                    n123 = for {
                      shift-right: [w352] -> w349
                      shift-left: w348 -> [w353]
                      tunnel: string[] ["STOP", "RESET ENCODERS", "RESET YAW", "ARDUINO MODE 0"] -> [w351] mode=indexing
                      n124 = Enqueue Element(queue=w353, element=w351) -> (queue out=w352:refnum<queue>)  [unwired: 2 in, 2 out]
                    }
                  }
                }
              }
              frame 10 {
                n125 = Dequeue Element(queue=w366, timeout in ms (-1)=w365, error in (no error)=w364) -> (element=w355:T9)  [unwired: 3 out]
                n126 = Greater?(x=w363, y=150.0) -> (0:w360:bool)
                n127 = Or(x=w360, y=w361) -> (x .or. y?=w356:bool)
                n128 = case shown="\"Exit\"" w355 {
                  tunnel: w356 -> [w369 _]
                  tunnel: [w373 State_Type_Definitions,_for_0.26g_versions_and_later_2."True Stop" ("Enum")] -> w357
                  tunnel: w359 -> [w370 w389]
                  tunnel: [w368 w388] -> w358
                  tunnel: [State_Type_Definitions,_for_0.26g_versions_and_later_2."Idle" ("Enum") State_Type_Definitions,_for_0.26g_versions_and_later_2."Shutdown" ("Enum")] -> w354
                  frame "None", Default {
                    n129 = case shown="False" w369 {
                      tunnel: w370 -> [w376 w382]
                      tunnel: [w375 w380] -> w368
                      frame False {
                        n130 = for {
                          shift-right: [w378] -> w375
                          shift-left: w376 -> [w379]
                          tunnel: string[] ["READ ENCODERS", "R-ACW"] ("element") -> [w377] mode=indexing
                          n131 = Enqueue Element(queue=w379, element=w377) -> (queue out=w378:refnum<queue>)  [unwired: 2 in, 2 out]
                        }
                      }
                      frame True {
                        n132 = for {
                          shift-right: [w384] -> w380
                          shift-left: w382 -> [w385]
                          tunnel: string[] ["RESET YAW", "RESET ENCODERS", "STOP", "ARDUINO MODE 0"] -> [w383] mode=indexing
                          n133 = Enqueue Element(queue=w385, element=w383) -> (queue out=w384:refnum<queue>)  [unwired: 2 in, 2 out]
                        }
                      }
                    }
                    n134 = Select(t=State_Type_Definitions,_for_0.26g_versions_and_later_2."True Stop" ("Enum"), s=w369, f=State_Type_Definitions,_for_0.26g_versions_and_later_2."Task 3" ("Enum")) -> (s? t:f=w373:T8)
                  }
                  frame "Exit" {
                    n135 = for {
                      shift-right: [w392] -> w388
                      shift-left: w389 -> [w393]
                      tunnel: string[] ["STOP", "RESET ENCODERS", "RESET YAW", ""] -> [w391] mode=indexing
                      n136 = Enqueue Element(queue=w393, element=w391) -> (queue out=w392:refnum<queue>)  [unwired: 2 in, 2 out]
                    }
                  }
                }
              }
              frame 11 {
                w398 = 20
                # ">> Outputs true if object detected >>"
                # ">> Manual override >>"
                n137 = Dequeue Element(queue=w407, timeout in ms (-1)=w406, error in (no error)=w405) -> (element=w404:T9)  [unwired: 3 out]
                n138 = Less?(x=w400, y=w398) -> (x < y?=w396:bool)
                n139 = Less?(x=w399, y=w398) -> (x < y?=w397:bool)
                n140 = And(x=w397, y=w396) -> (x .and. y?=w395:bool)
                "Detect?" <- w395
                n141 = case shown="\"None\", Default" w404 {
                  tunnel: [w417 State_Type_Definitions,_for_0.26g_versions_and_later_2."True Stop" ("Enum")] -> w403
                  tunnel: [w415 w436] -> w402
                  tunnel: w408 -> [w414 _]
                  tunnel: w401 -> [w412 _]
                  tunnel: w395 -> [w410 _]
                  tunnel: [w409 State_Type_Definitions,_for_0.26g_versions_and_later_2."Shutdown" ("Enum")] -> w394
                  frame "None", Default {
                    # ">> WIill proceed to part ii if not manual override >>"
                    # ">>If ENABLE or Trigger is set to true>>"
                    n142 = Or(x=w410, y=w412) -> (x .or. y?=w411:bool)
                    n143 = case shown="False" w411 {
                      tunnel: [w424 w429] -> w415
                      tunnel: w414 -> [w422 w428]
                      frame False {
                        n144 = for {
                          shift-right: [w426] -> w424
                          shift-left: w422 -> [w427]
                          tunnel: string[] ["FORWARD", "ULTRASONIC READ", ""] ("element") -> [w425] mode=indexing
                          n145 = Enqueue Element(queue=w427, element=w425) -> (queue out=w426:refnum<queue>)  [unwired: 2 in, 2 out]
                        }
                      }
                      frame True {
                        n146 = for {
                          shift-right: [w432] -> w429
                          shift-left: w428 -> [w433]
                          tunnel: string[] ["STOP", "RESET ENCODERS", "RESET YAW", "ARDUINO MODE 0"] -> [w431] mode=indexing
                          n147 = Enqueue Element(queue=w433, element=w431) -> (queue out=w432:refnum<queue>)  [unwired: 2 in, 2 out]
                        }
                      }
                    }
                    n148 = case shown="False" w412 {
                      tunnel: [State_Type_Definitions,_for_0.26g_versions_and_later_2."True Stop" ("Enum") State_Type_Definitions,_for_0.26g_versions_and_later_2."True Stop" ("Enum")] -> w413
                      tunnel: [State_Type_Definitions,_for_0.26g_versions_and_later_2."Task 4_B" ("Enum") State_Type_Definitions,_for_0.26g_versions_and_later_2."Idle" ("Enum")] -> w409
                      frame False {
                      }
                      frame True {
                      }
                    }
                    n149 = Select(t=w413, s=w411, f=State_Type_Definitions,_for_0.26g_versions_and_later_2."Task 4_A" ("Enum")) -> (s? t:f=w417:T8)
                  }
                  frame "Exit" {
                    n150 = for {
                      shift-right: [w439] -> w436
                      shift-left: _ -> [w440]
                      tunnel: string[] ["STOP", "RESET ENCODERS", "RESET YAW", ""] -> [w438] mode=indexing
                      n151 = Enqueue Element(queue=w440, element=w438) -> (queue out=w439:refnum<queue>)  [unwired: 2 in, 2 out]
                    }
                  }
                }
              }
              frame 12 {
                w451 = 20
                # ">> Outputs true if 150 mm has been moved >>"
                # ">> Outputs true if sensor not obstructed>>"
                # ">> Manual override >>"
                n152 = Dequeue Element(queue=w456, timeout in ms (-1)=w455, error in (no error)=w454) -> (element=w453:T9)  [unwired: 3 out]
                n153 = Greater?(x=w448, y=w451) -> (0:w449:bool)
                n154 = Greater?(x=w447, y=w451) -> (0:w450:bool)
                n155 = Greater Or Equal?(x=w443, y=80.0) -> (x >= y?=w445:bool)
                n156 = And(x=w450, y=w449) -> (x .and. y?=w444:bool)
                n157 = And(x=w445, y=w444) -> (x .and. y?=w441:bool)
                n158 = case shown="\"None\", Default" w453 {
                  tunnel: [w468 State_Type_Definitions,_for_0.26g_versions_and_later_2."True Stop" ("Enum")] -> w458
                  tunnel: [w466 w487] -> w459
                  tunnel: w452 -> [w465 _]
                  tunnel: w457 -> [w463 _]
                  tunnel: w441 -> [w461 _]
                  tunnel: [w460 State_Type_Definitions,_for_0.26g_versions_and_later_2."Shutdown" ("Enum")] -> w442
                  frame "None", Default {
                    # ">> WIill proceed to part ii if not manual override >>"
                    # ">>If ENABLE or Trigger is set to true>>"
                    n159 = Or(x=w461, y=w463) -> (x .or. y?=w462:bool)
                    n160 = case shown="False" w462 {
                      tunnel: [w475 w480] -> w466
                      tunnel: w465 -> [w473 w479]
                      frame False {
                        n161 = for {
                          shift-right: [w477] -> w475
                          shift-left: w473 -> [w478]
                          tunnel: string[] ["RIGHT", "ULTRASONIC READ", "READ ENCODERS"] ("element") -> [w476] mode=indexing
                          n162 = Enqueue Element(queue=w478, element=w476) -> (queue out=w477:refnum<queue>)  [unwired: 2 in, 2 out]
                        }
                      }
                      frame True {
                        n163 = for {
                          shift-right: [w483] -> w480
                          shift-left: w479 -> [w484]
                          tunnel: string[] ["STOP", "RESET ENCODERS", "RESET YAW", "ARDUINO MODE 0"] -> [w482] mode=indexing
                          n164 = Enqueue Element(queue=w484, element=w482) -> (queue out=w483:refnum<queue>)  [unwired: 2 in, 2 out]
                        }
                      }
                    }
                    n165 = case shown="True" w463 {
                      tunnel: [State_Type_Definitions,_for_0.26g_versions_and_later_2."True Stop" ("Enum") State_Type_Definitions,_for_0.26g_versions_and_later_2."True Stop" ("Enum")] -> w464
                      tunnel: [State_Type_Definitions,_for_0.26g_versions_and_later_2."Task 4_C" ("Enum") State_Type_Definitions,_for_0.26g_versions_and_later_2."Idle" ("Enum")] -> w460
                      frame False {
                      }
                      frame True {
                      }
                    }
                    n166 = Select(t=w464, s=w462, f=State_Type_Definitions,_for_0.26g_versions_and_later_2."Task 4_B" ("Enum")) -> (s? t:f=w468:T8)
                  }
                  frame "Exit" {
                    n167 = for {
                      shift-right: [w490] -> w487
                      shift-left: _ -> [w491]
                      tunnel: string[] ["STOP", "RESET ENCODERS", "RESET YAW", ""] -> [w489] mode=indexing
                      n168 = Enqueue Element(queue=w491, element=w489) -> (queue out=w490:refnum<queue>)  [unwired: 2 in, 2 out]
                    }
                  }
                }
              }
              frame 13 {
                w506 = 20
                # ">> Outputs true if object detected >>"
                # ">> Manual override >>"
                n169 = Dequeue Element(queue=w501, timeout in ms (-1)=w493, error in (no error)=w492) -> (element=w494:T9)  [unwired: 3 out]
                n170 = Less?(x=w502, y=w506) -> (x < y?=w504:bool)
                n171 = Less?(x=w503, y=w506) -> (x < y?=w505:bool)
                n172 = And(x=w505, y=w504) -> (x .and. y?=w499:bool)
                n173 = case shown="\"None\", Default" w494 {
                  tunnel: [w515 State_Type_Definitions,_for_0.26g_versions_and_later_2."True Stop" ("Enum")] -> w497
                  tunnel: [w513 w535] -> w496
                  tunnel: w500 -> [w512 w532]
                  tunnel: w498 -> [w510 _]
                  tunnel: w499 -> [w508 _]
                  tunnel: [w507 State_Type_Definitions,_for_0.26g_versions_and_later_2."Shutdown" ("Enum")] -> w495
                  frame "None", Default {
                    # ">> WIill proceed to part ii if not manual override >>"
                    # ">>If ENABLE or Trigger is set to true>>"
                    n174 = Or(x=w508, y=w510) -> (x .or. y?=w509:bool)
                    n175 = case shown="False" w509 {
                      tunnel: [w522 w527] -> w513
                      tunnel: w512 -> [w520 w526]
                      frame False {
                        n176 = for {
                          shift-right: [w524] -> w522
                          shift-left: w520 -> [w525]
                          tunnel: string[] ["FORWARD", "ULTRASONIC READ", ""] ("element") -> [w523] mode=indexing
                          n177 = Enqueue Element(queue=w525, element=w523) -> (queue out=w524:refnum<queue>)  [unwired: 2 in, 2 out]
                        }
                      }
                      frame True {
                        n178 = for {
                          shift-right: [w530] -> w527
                          shift-left: w526 -> [w531]
                          tunnel: string[] ["STOP", "RESET ENCODERS", "RESET YAW", "ARDUINO MODE 0"] -> [w529] mode=indexing
                          n179 = Enqueue Element(queue=w531, element=w529) -> (queue out=w530:refnum<queue>)  [unwired: 2 in, 2 out]
                        }
                      }
                    }
                    n180 = case shown="True" w510 {
                      tunnel: [State_Type_Definitions,_for_0.26g_versions_and_later_2."True Stop" ("Enum") State_Type_Definitions,_for_0.26g_versions_and_later_2."True Stop" ("Enum")] -> w511
                      tunnel: [State_Type_Definitions,_for_0.26g_versions_and_later_2."Idle" ("Enum") State_Type_Definitions,_for_0.26g_versions_and_later_2."Idle" ("Enum")] -> w507
                      frame False {
                      }
                      frame True {
                      }
                    }
                    n181 = Select(t=w511, s=w509, f=State_Type_Definitions,_for_0.26g_versions_and_later_2."Task 4_C" ("Enum")) -> (s? t:f=w515:T8)
                  }
                  frame "Exit" {
                    n182 = for {
                      shift-right: [w538] -> w535
                      shift-left: w532 -> [w539]
                      tunnel: string[] ["STOP", "RESET ENCODERS", "RESET YAW", ""] -> [w537] mode=indexing
                      n183 = Enqueue Element(queue=w539, element=w537) -> (queue out=w538:refnum<queue>)  [unwired: 2 in, 2 out]
                    }
                  }
                }
              }
            }
          }
        }
        n184 = local write "Green LED"(w133) -> ()
      }
      n185 = call <vilib>:"DIO Close.vi"("error in (no error)"=w7, "DIO Info In"=w10) -> ()  [unwired: 9 in, 1 out]
      n186 = call <vilib>:"DIO Close.vi"("error in (no error)"=w17, "DIO Info In"=w19) -> ()  [unwired: 9 in, 1 out]
      n187 = call <vilib>:"NavX Close.vi"("error in (no error)"=w5, "NavX Info In"=w6) -> ()  [unwired: 9 in, 1 out]
      n188 = call <vilib>:"DIO Close.vi"("error in (no error)"=w12, "DIO Info In"=w14) -> ()  [unwired: 9 in, 1 out]
      n189 = Merge Errors "Merge Errors"(w47, w46) -> (w29:errorcluster)
      n190 = Merge Errors(w33, w29) -> (w28:errorcluster)
      n191 = Destroy User Event(user event=w50, error in=w28) -> ()  [unwired: 1 out]
      n192 = Destroy User Event(user event=w51, error in=w28) -> ()  [unwired: 1 out]
      n193 = Unregister For Events(event registration refnum=w42, error in=w28) -> ()  [unwired: 1 out]
      n194 = Release Queue(queue=w24, error in (no error)=w28) -> (error out=w4:errorcluster)  [unwired: 1 in, 2 out]
      n195 = Release Queue(queue=w41, error in (no error)=w28) -> ()  [unwired: 1 in, 3 out]
      n196 = call <vilib>:"Simple Error Handler.vi"("error in (no error)"=w4) -> ("error out"=w3:errorcluster)  [unwired: 4 in, 4 out]
      n197 = call <vilib>:"Reset myRIO.vi"("error in (no error)"=w3) -> ("error out"=→"error out":errorcluster)  [unwired: 10 in]
    }
    frame #2 {
      n198 = Wait (ms)(milliseconds to wait=u32 100) -> ()  [unwired: 1 out]
    }
  }
